vi "Create Test Configuration.vi"() -> (0 "error out":errorcluster, 1 "Names":string[](array[string]), 2 "Line Array":T1[](array[typedef]), 3 "Module Configuration":refnum<class "Benchmark PID configuration.lvclass">, 4 "Channels":refnum<class "TBM channel.lvclass">[](array[class]), 5 "instance identifier":string)   [LabVIEW 2018, in "Benchmark PID tests.lvlib"]
doc: "This VI creates a standard test configuration for other unit tests. It currently creates and adds one line with every datatype to the module configuration."
uses:
  Benchmark PID tests.lvlib
  module/configuration/Benchmark PID configuration.lvclass
  C:/Program Files (x86)/National Instruments/LabVIEW 2018/vi.lib/NI/Configuration Framework/serializable configuration/NISE_CEF_serializable configuration.lvclass
  module/configuration/Line.ctl
  <vilib>/NI/Tag Bus Module Framework/channel/TBM channel.lvclass
  <vilib>/NI/Configuration Framework/serializable configuration/NISE_CEF_serializable configuration.lvclass
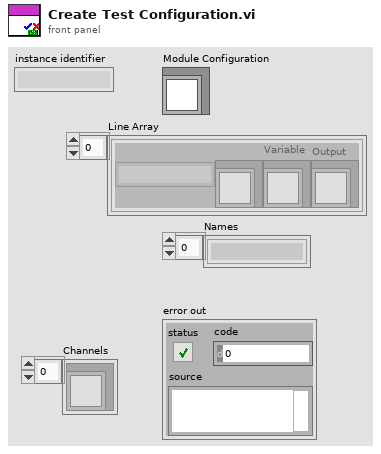
[diagram p1: front panel]
types:
  T1 = typedef "Benchmark PID configuration.lvclass/Line.ctl" = cluster{"PID Name":string, "Setpoint":refnum<class "TBM channel.lvclass">, "Variable":refnum<class "TBM channel.lvclass">, "Output":refnum<class "TBM channel.lvclass">}
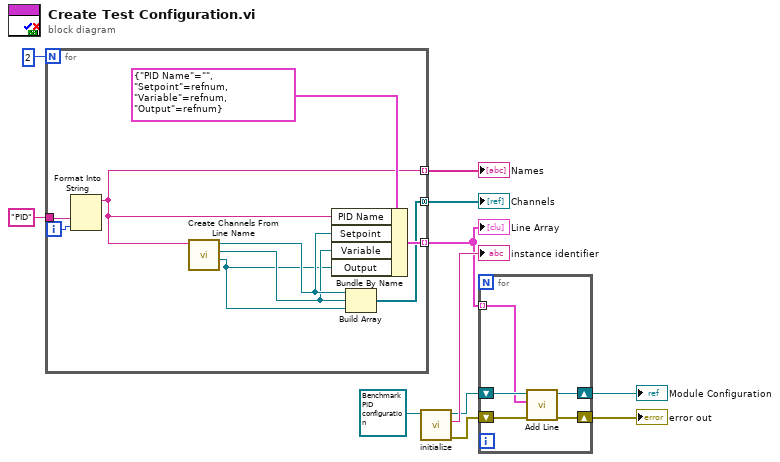
[diagram p0: block diagram]
diagram:
  n1 = for {
    N: 2 -> [_]
    tunnel: [w18] -> w7 mode=indexing
    tunnel: [w16] -> w1 mode=concatenating
    tunnel: [w12] -> w8 mode=indexing
    tunnel: "PID" -> [w17]
    i -> [w19]
    n2 = Format Into String(w17, w19) -> (resulting string=w12:string)  [unwired: 3 in, 1 out]
    n3 = call "Create Channels From Line Name.vi"("String"=w12) -> ("channel"=w13:refnum<class "TBM channel.lvclass">, "channel 2"=w14:refnum<class "TBM channel.lvclass">, "TBM channel out"=w15:refnum<class "TBM channel.lvclass">)  [unwired: 8 in]
    n4 = Bundle By Name(cluster=T1 {"PID Name"="", "Setpoint"=refnum, "Variable"=refnum, "Output"=refnum} ("Line"), "PID Name"=w12, "Setpoint"=w15, "Variable"=w14, "Output"=w13) -> (w18:T1)
    n5 = Build Array(w15, w14, w13) -> (w16:refnum<class "TBM channel.lvclass">[])
  }
  "Names" <- w8
  "Line Array" <- w7
  "Channels" <- w1
  n6 = call <vilib>:"initialize.vi"("configuration in"=refnum<class "Benchmark PID configuration.lvclass"> refnum ("tag bus configurable plugin module configuration")) -> ("error out"=w9:errorcluster, "identifier"=→"instance identifier":string, "configuration out"=w4:refnum<class "Benchmark PID configuration.lvclass">)  [unwired: 8 in]
  n7 = for {
    tunnel: w7 -> [w21] mode=indexing
    shift-right: [w24] -> w6
    shift-left: w4 -> [w25]
    shift-right: [w22] -> w11
    shift-left: w9 -> [w23]
    n8 = call "Add Line.vi"("error in"=w23, "Line"=w21, "Benchmark PID configuration in"=w25) -> ("error out"=w22:errorcluster, "Benchmark PID configuration out"=w24:refnum<class "Benchmark PID configuration.lvclass">)  [unwired: 6 in, 1 out]
  }
  "error out" <- w11
  "Module Configuration" <- w6
